vi "preguntaSimulacion.vi"(2 "error in (no error)":errorcluster) -> (0 "error out":errorcluster, 1 "Sim":bool)   [LabVIEW 2019, in "Prueba.lvclass"]
uses:
  Prueba.lvclass
panel:
  out "simular?":string
  in  "no":bool
  in  "si":bool
  # "¿Simular Instrumentos?"
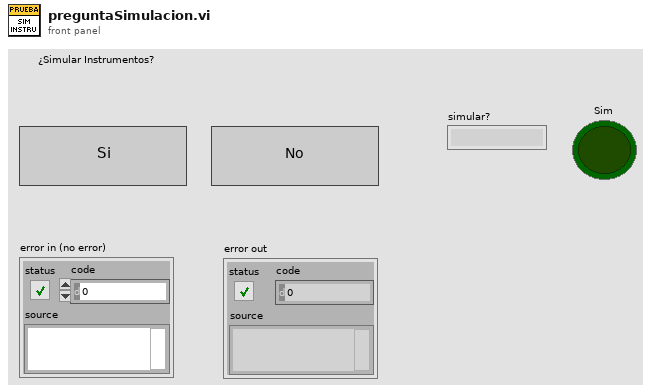
[diagram p1: front panel]
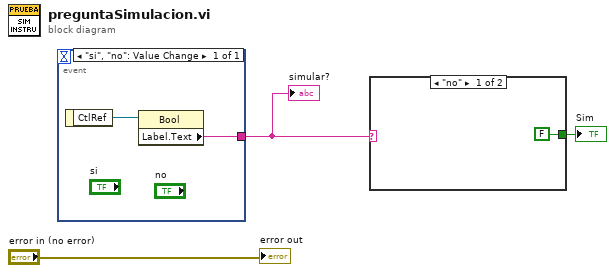
[diagram p0: block diagram]
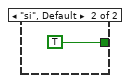
[diagram p2: hidden frame]
diagram:
  n1 = event shown="[0] \"si\", \"no\": Value Change" {
    selector: _ -> [_]
    dyn-events: _ -> [_]
    timeout: _ -> [_]
    tunnel: [w4] -> w2
    event "si", "no": Value Change {
      n2 = event-data() -> ("CtlRef"=w5:refnum<vi>)  [unwired: 1 in]
      n3 = property class="Bool"(reference=w5) -> ("Label.Text"=w4:string)  [unwired: 1 in, 2 out]
    }
  }
  "simular?" <- w2
  n4 = case shown="\"no\"" w2 {
    tunnel: [FALSE TRUE] -> w1
    frame "no" {
    }
    frame "si", Default {
    }
  }
  "Sim" <- w1
  "error out" <- "error in (no error)"
